vi "New.vi"(8 "error in (no error)":errorcluster, 11 "reference in":refnum<class "Test_Flux_Capacitor.lvclass">) -> (0 "error out":errorcluster, 3 "reference out":refnum<class "Test_Flux_Capacitor.lvclass">)   [LabVIEW 2022 SP3, in "Test_Flux_Capacitor.lvlib" / "Test_Flux_Capacitor.lvclass"]
uses:
  Test_Flux_Capacitor.lvclass
  ObjectAttributes.ctl
  Components/DMM_Keysight_34980A.lvlibp/DMM_Keysight_34980A.lvclass
  Components/LCR_BK891.lvlibp/LCR_BK891.lvclass
  Components/PSU_Base.lvlibp/PSU_Base.lvclass
  Components/SwitchBase.lvlibp/SwitchBase.lvclass
  Components/Flux_Capacitor.lvlibp/Flux_Capacitor.lvclass
  Components/Frequency_Counter_Base.lvlibp/Frequency_Counter_Base.lvclass
  Components/JTAG_Base.lvlibp/JTAG_Base.lvclass
  Config.ctl
  Test_Flux_Capacitor.lvclass/Test_Flux_Capacitor.ctl
  Components/Test_Base.lvlibp/Test_Base.lvclass
panel:
  in  "Data":T1
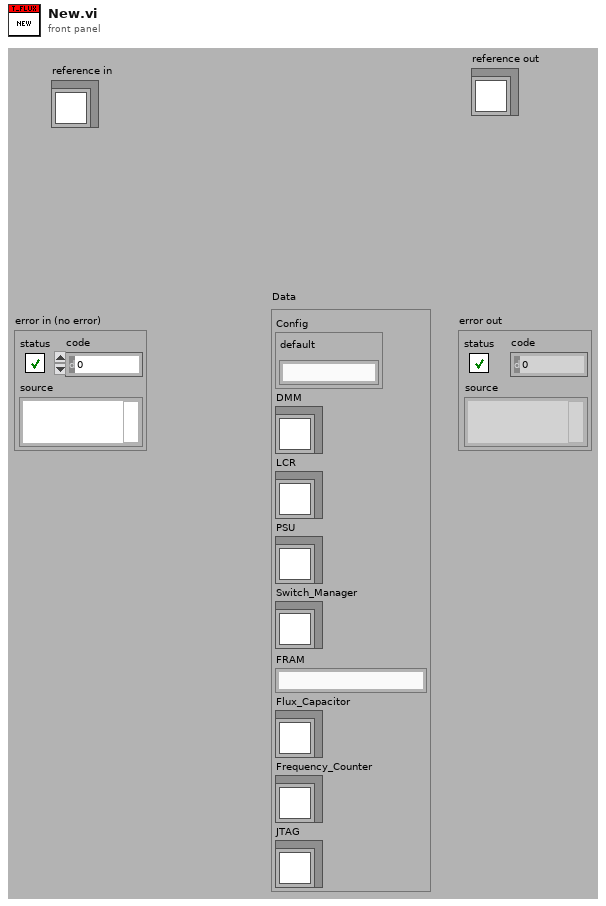
[diagram p1: front panel]
types:
  T1 = typedef "Test_Flux_Capacitor.lvlib/Test_Flux_Capacitor.lvclass/ObjectAttributes.ctl" = cluster{"Config":T2, "DMM":refnum<class "DMM_Keysight_34980A.lvclass">, "LCR":refnum<class "LCR_BK891.lvclass">, "PSU":refnum<class "PSU_Base.lvclass">, "Switch_Manager":refnum<class "SwitchBase.lvclass">, "FRAM":string, "Flux_Capacitor":refnum<class "Flux_Capacitor.lvclass">, "Frequency_Counter":refnum<class "Frequency_Counter_Base.lvclass">, "JTAG":refnum<class "JTAG_Base.lvclass">}
  T2 = typedef "Test_Flux_Capacitor.lvlib/Test_Flux_Capacitor.lvclass/Config.ctl" = cluster{"default":string}
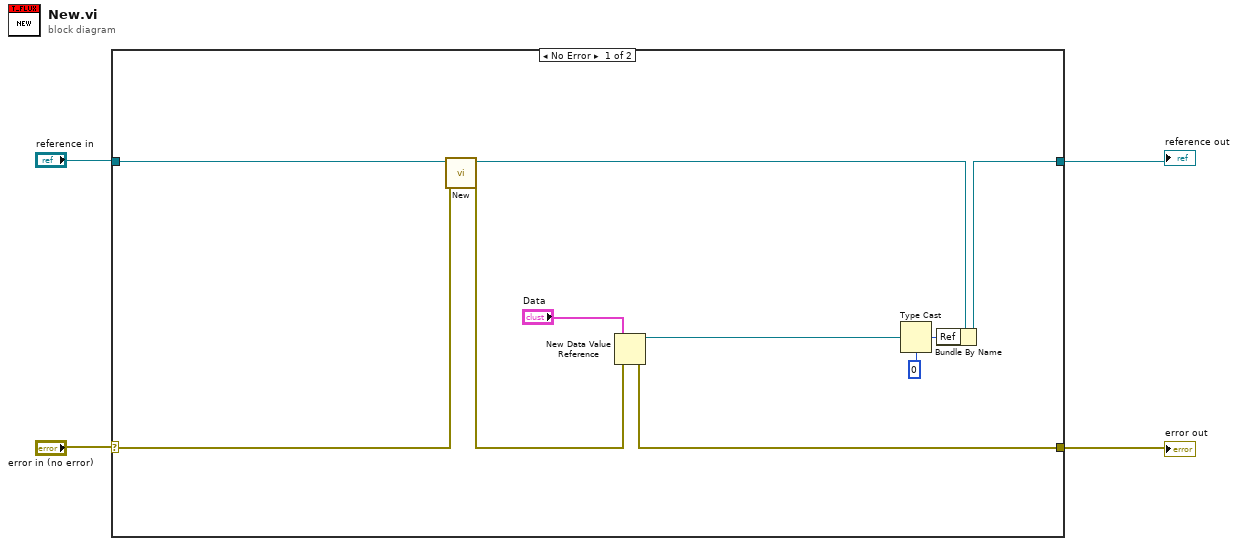
[diagram p0: block diagram]
diagram:
  n1 = case shown="No Error" "error in (no error)" {
    selector: "error in (no error)" -> [w8 w16]
    tunnel: [w6 w16] -> w2
    tunnel: "reference in" -> [w14 w15]
    tunnel: [w13 w15] -> w1
    frame No Error {
      n2 = call-parent "New.vi"("error in (no error)"=w8, "reference in"=w14) -> ("error out"=w7:errorcluster, "reference out"=w12:refnum<class "Test_Flux_Capacitor.lvclass">)  [unwired: 8 in]
      n3 = New Data Value Reference(data value="Data", error in=w7) -> (data value reference=w10:refnum<data-value>, error out=w6:errorcluster)
      n4 = Type Cast(type=u32 0 ("DataRef"), x=w10) -> (*(type *) &x=w9:u32)
      n5 = Bundle By Name(cluster=w12, "Ref"=w9) -> (w13:refnum<class "Test_Flux_Capacitor.lvclass">)
    }
    frame Error {
    }
  }
  "error out" <- w2
  "reference out" <- w1
